vi "Mcp2210 Open By SN.vi"(6 "devPathsize":u32, 7 "devPath":u16, 9 "serialNo":u16, 10 "pid":u16, 11 "vid":u16) -> (1 "serialNo out":u16, 3 "function return":u32, 4 "devPathsize out":u32, 5 "devPath out":u16)   [LabVIEW 2015, in "mcp2210.lvlib"]
doc: "Opens the connection with the MCP2210 device identified by the given VID:PID\nand the serial number string and returns the file handle.\nAlso, the function can provide the device path as NULL terminated UNICODE string, if a valid pointer\nto a buffer of sufficient size is provisioned. If the buffer size is smaller than required,\nthe function call fails, the device is not opened, but the devPathsize parameter contains the value\nrequired for the path string size.\nThe function provides also the option to skip the path string if this is not needed.\n!!! Important note !!!\nIn case of failure, the function returns an invalid handle value (-1) and updates an internal variable\nwith the specific error code (negative values). This can be retrieved with Mcp2210_GetLastError() call.\nThe error codes that Mcp2210_GetLastError() might return after Mcp2210_OpenBySN() call are:\n- E_SUCCESS (0), if no error occurred\n- E_ERR_BUFFER_TOO_SMALL\n- E_ERR_UNKOWN_ERROR, E_ERR_MALLOC, E_ERR_NULL,\nE_ERR_DEVICE_NOT_FOUND, E_ERR_NO_SUCH_SERIALNR,\nE_ERR_CONNECTION_ALREADY_OPENED, E_ERR_OPEN_DEVICE_ERROR\nParameters:\nInputs:\n- unsigned short vid - MCP2210 device VendorID (Microchip default = 0x4D8)\n- unsigned short pid - MCP2210 device ProductID (Microchip default = 0xDE)\n- wchar_t *serialNo - The serial number of the MCP2210 we want to connect to:\nNULL terminated string of max MPC2210_SERIAL_NUMBER_LENGTH wide\ncharacters\nCannot be NULL.\n- unsigned long *devPathsize - pointer to the variable that contains the size of the buffer\nin which the device path must be copied. The size is expressed\nin bytes and must accommodate also the string NULL terminator.\nIf the pointer is NULL, or if the *devPathsize is 0, the path\nis not returned and the *devPath parameter is ignored.\nOutputs:\n- wchar_t *devPath - path string buffer pointer.\nIf *devPath pointer is NULL, the path is not reported,\n*devPathsize parameter is ignored, but the device is opened\nand the function returns the handle.\n- unsigned long *devPathsize - if the function call fails because of insufficient buffer size\n(Mcp2210_GetLastError() returns E_ERR_BUFFER_TOO_SMALL), this\nparameter indicates the necessary buffer size to accommodate the\npath string size (in bytes).\nReturns:\n- valid handle value in case of success\n- INVALID_HANDLE_VALUE (-1) in case of error.\n\nMCP2210_DLL_UM_API void* __stdcall Mcp2210_OpenBySN(unsigned short vid, unsigned short pid, unsigned short *serialNo, unsigned short *devPath, unsigned long *devPathsize);"
uses:
  <userlib>/mcp2210/mcp2210.lvlib
  <userlib>/mcp2210/mcp2210_dll_um_x86.dll
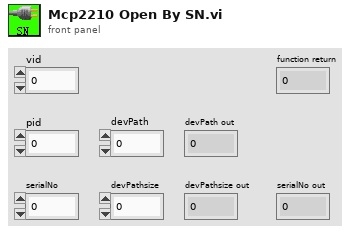
[diagram p1: front panel]
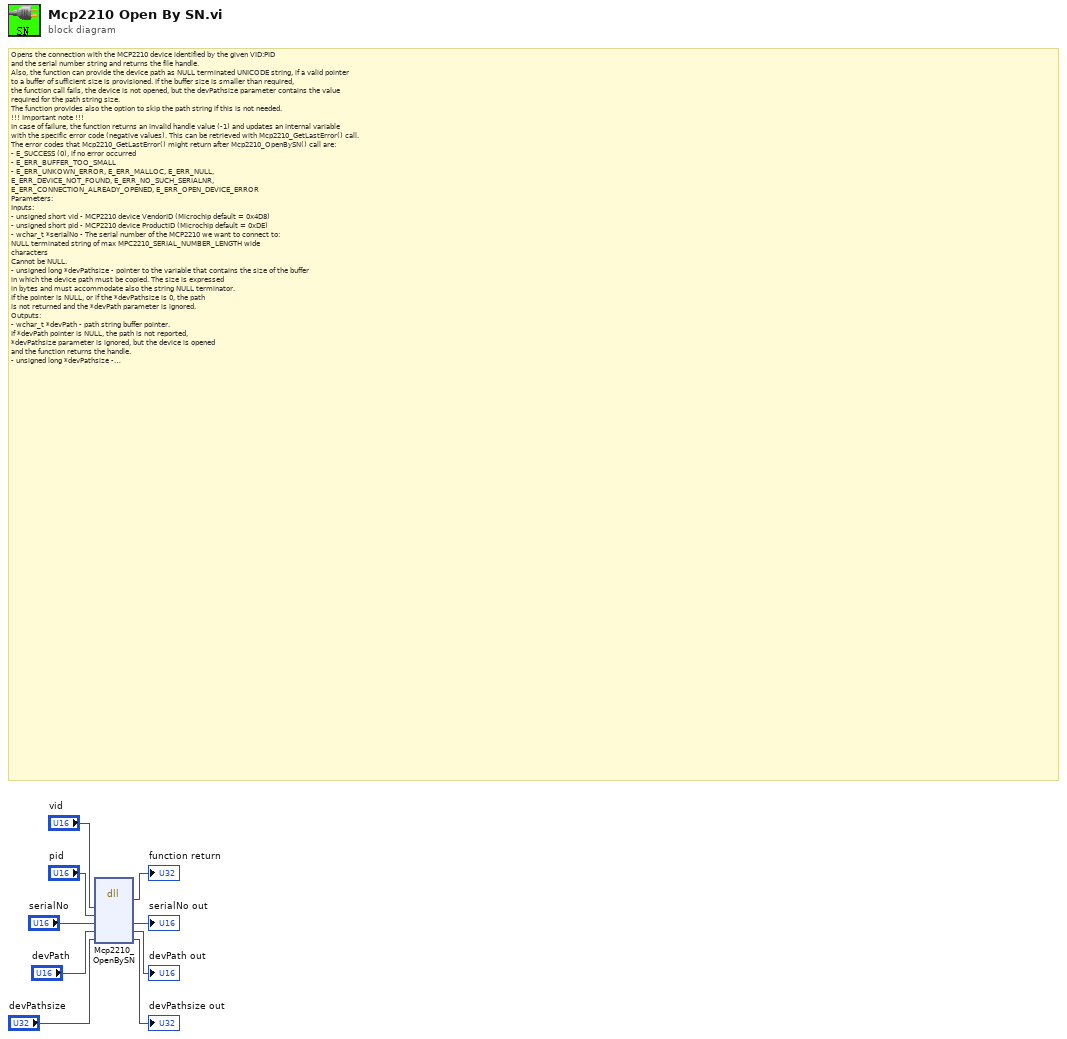
[diagram p0: block diagram]
diagram:
  # "Opens the connection with the MCP2210 device identified by the given VID:PID\nand the serial number string and returns the file handle.\nAlso, the function can provide the device path as NULL terminated UNICODE string, if a valid pointer\nto a buffer of sufficient size is provisioned. If the buffer size is smaller than required,\nthe function call fails, the device is not opened, but the devPathsize parameter contains the value\nrequired for the path string size.\nThe function provides also the option to skip the path string if this is not needed.\n!!! Important note !!!\nIn case of failure, the function returns an invalid handle value (-1) and updates an internal variable\nwith the specific error code (negative values). This can be retrieved with Mcp2210_GetLastError() call.\nThe error codes that Mcp2210_GetLastError() might return after Mcp2210_OpenBySN() call are:\n- E_SUCCESS (0), if no error occurred\n- E_ERR_BUFFER_TOO_SMALL\n- E_ERR_UNKOWN_ERROR, E_ERR_MALLOC, E_ERR_NULL,\nE_ERR_DEVICE_NOT_FOUND, E_ERR_NO_SUCH_SERIALNR,\nE_ERR_CONNECTION_ALREADY_OPENED, E_ERR_OPEN_DEVICE_ERROR\nParameters:\nInputs:\n- unsigned short vid - MCP2210 device VendorID (Microchip default = 0x4D8)\n- unsigned short pid - MCP2210 device ProductID (Microchip default = 0xDE)\n- wchar_t *serialNo - The serial number of the MCP2210 we want to connect to:\nNULL terminated string of max MPC2210_SERIAL_NUMBER_LENGTH wide\ncharacters\nCannot be NULL.\n- unsigned long *devPathsize - pointer to the variable that contains the size of the buffer\nin which the device path must be copied. The size is expressed\nin bytes and must accommodate also the string NULL terminator.\nIf the pointer is NULL, or if the *devPathsize is 0, the path\nis not returned and the *devPath parameter is ignored.\nOutputs:\n- wchar_t *devPath - path string buffer pointer.\nIf *devPath pointer is NULL, the path is not reported,\n*devPathsize parameter is ignored, but the device is opened\nand the function returns the handle.\n- unsigned long *devPathsize - if the function call fails because of insufficient buffer size\n(Mcp2210_GetLastError() returns E_ERR_BUFFER_TOO_SMALL), this\nparameter indicates the necessary buffer size to accommodate the\npath string size (in bytes).\nReturns:\n- valid handle value in case of success\n- INVALID_HANDLE_VALUE (-1) in case of error.\n\nMCP2210_DLL_UM_API void* __stdcall Mcp2210_OpenBySN(unsigned short vid, unsigned short pid, unsigned short *serialNo, unsigned short *devPath, unsigned long *devPathsize);"
  n1 = dll-call lib="D:/LabVIEW 2015/user.lib/mcp2210/mcp2210_dll_um_x86.*" fn="Mcp2210_OpenBySN"("vid"="vid", "pid"="pid", "serialNo"="serialNo", "devPath"="devPath", "devPathsize"="devPathsize") -> (→"function return":u32, "serialNo"=→"serialNo out":u16, "devPath"=→"devPath out":u16, "devPathsize"=→"devPathsize out":u32)  [unwired: 5 in, 2 out]
